vi "MT MSK Mod-Demod.vi"() -> ()   [LabVIEW 2010]
doc: "This example demonstrates the programming of an MSK Modulation Demodulation System."
uses:
  <vilib>/addons/Modulation/Digital/General/MT Generate Bits (Galois, PN Order).vi
  <vilib>/AddOns/Modulation/Digital/General/MT Generate MSK System Parameters.vi
  <vilib>/AddOns/Modulation/Digital/General/MT Apply Matched Filter (MSK).vi
  <vilib>/AddOns/Modulation/Digital/General/MT Align To Ideal Symbols (MSK).vi
  <vilib>/AddOns/Modulation/Digital/General/MT Map MSK Symbols to Bits.vi
  <vilib>/AddOns/Modulation/Digital/Demodulation/MT Calculate BER After Trigger (PN Sequence).vi
  <vilib>/addons/Modulation/niDMT.lvlib
panel:
  in  "autoscale":bool
  out "Constellation Graph, RX (in)":T1(graph)
  out "Recovered Message Bits":i8[](array[numeric])
  in  "Differential Encoding Enable":enum16{"disable", "enable"}(ring)
  in  "Seed In":i32=-1
  out "error out":errorcluster
  in  "stop":bool
  out "BER":dbl format="%.4f"
  in  "PN Sequence Order":i32=9
  in  "Reset? (T)":bool=TRUE
  in  "Eb/N0 (dB)":dbl(slide)=50.0 scale=0.0..100.0
  in  "Symbol Rate (Hz)":dbl=400000.0 format="%.2p"
  in  "Pulse Shaping Filter":T2(ring)=enum."Gaussian"
  in  "MSK Symbols":i32=1000
  in  "Samples per Symbol":i32=16
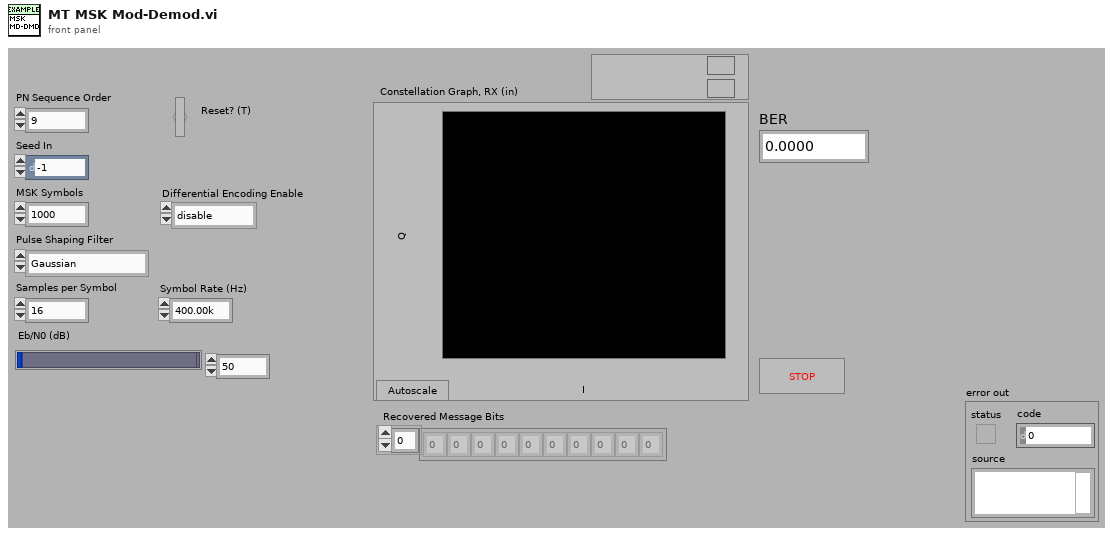
[diagram p1: front panel]
types:
  T1 = cluster{"Decimated Array":dbl[], "Decimated Array":dbl[]}[]
  T2 = enum16{"none", "Raised Cosine", "Root Raised Cos", "Gaussian"}
  T3 = enum16{"FSK", "PSK", "QAM", "MSK", "PAM", "ASK", "CPM"}
  T4 = cluster{"differential encoding enable":enum16{"disable", "enable"}, "samples per symbol (16)":i32}
  T5 = typedef "niAMT.lvlib/Complex Data Waveform.ctl" = cluster{"t0":dbl, "dt":dbl, "Y":cdb[]}
  T6 = cluster{"constellation":dbl[], "oversampled data":dbl[]}[]
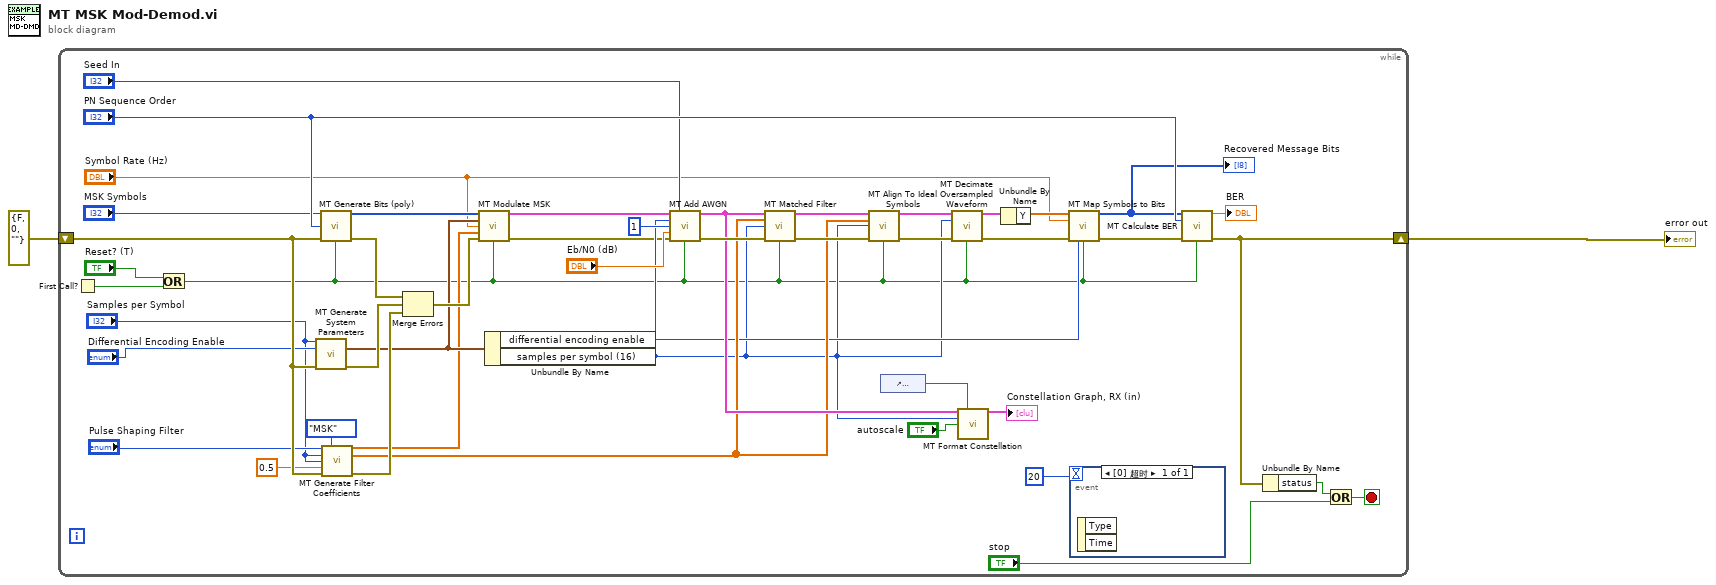
[diagram p0: block diagram]
diagram:
  n1 = while {
    shift-right: [w38] -> w2
    shift-left: errorcluster {"status"=FALSE, "code"=0, "source"=""} ("error out") -> [w49]
    stop <- w37 stop-if-true
    n2 = First Call?() -> (First Call?: T/F=w28:bool)
    n3 = Or(x="Reset? (T)", y=w28) -> (x .or. y?=w6:bool)
    n4 = call-poly <vilib>:"MT Generate System Parameters.vi"("samples per symbol (16)"="Samples per Symbol", "differential encoding enable"="Differential Encoding Enable", "error in (no error)"=w49) -> ("MSK system parameters"=w10:T4, "error out"=w44:errorcluster)  [unwired: 2 in, 9 out]
    n5 = call-poly <vilib>:"MT Generate Bits (poly).vi"("total bits (128)"="MSK Symbols", "PN sequence order (9)"="PN Sequence Order", "error in (no error)"=w49, "reset? (T)"=w6) -> ("output bit stream"=w11:i8[], "error out"=w45:errorcluster)  [unwired: 1 in, 9 out]
    n6 = call <vilib>:"MT Generate Filter Coefficients.vi"("pulse shaping filter (none)"="Pulse Shaping Filter", "modulation type"=T3."MSK", "pulse shaping samples per symbol (16)"="Samples per Symbol", "matched samples per symbol (16)"="Samples per Symbol", "filter parameter"=0.5, "error in (no error)"=w49) -> ("pulse shaping filter coefficients"=w8:dbl[], "matched filter coefficients"=w19:dbl[], "error out"=w43:errorcluster)  [unwired: 1 in, 6 out]
    n7 = Merge Errors(w45, w44, w43) -> (w48:errorcluster)
    n8 = call <vilib>:"MT Modulate MSK.vi"("input bit stream"=w11, "MSK system parameters"=w10, "symbol rate (Hz)"="Symbol Rate (Hz)", "pulse shaping filter coefficients"=w8, "error in (no error)"=w48, "reset? (T)"=w6) -> ("output complex waveform"=w7:T5, "error out"=w5:errorcluster)  [unwired: 1 in, 7 out]
    n9 = Unbundle By Name(w10) -> ("differential encoding enable"=w14:enum16{"disable", "enable"}, "samples per symbol (16)"=w12:i32)
    n10 = call <vilib>:"MT Add AWGN.vi"("input complex waveform"=w7, "samples per symbol (16)"=w12, "bits per symbol (1)"=1, "Eb/N0 (10 dB)"="Eb/N0 (dB)", "error in (no error)"=w5, "seed in (0xFFFFFFFF)"="Seed In", "reset? (T)"=w6) -> ("output complex waveform"=w22:T5, "error out"=w27:errorcluster)  [unwired: 7 out]
    n11 = call-poly <vilib>:"MT Matched Filter.vi"("input complex waveform"=w22, "matched filter coefficients"=w19, "samples per symbol (16)"=w12, "error in (no error)"=w27, "reset? (T)"=w6) -> ("output phase waveform"=w20:cluster{"t0":dbl, "dt":dbl, "Y":dbl[]}, "error out"=w23:errorcluster)  [unwired: 9 out]
    n12 = call-poly <vilib>:"MT Align To Ideal Symbols.vi"("input phase waveform"=w20, "matched filter coefficients"=w19, "samples per symbol (16)"=w12, "error in (no error)"=w23, "reset? (T)"=w6) -> ("output phase waveform"=w17:cluster{"t0":dbl, "dt":dbl, "Y":dbl[]}, "error out"=w21:errorcluster)  [unwired: 9 out]
    n13 = control-ref of="Constellation Graph, RX (in)"() -> (w30:refnum<vi>)
    n14 = call <vilib>:"MT Decimate Oversampled Waveform.vi"("input complex waveform"=w17, "decimation factor"=w12, "error in (no error)"=w21, "reset? (T)"=w6) -> ("output complex waveform"=w16:T5, "error out"=w18:errorcluster)  [unwired: 1 in, 9 out]
    n15 = call <vilib>:"MT Format Constellation.vi"("waveform"=w22, "constellation reference"=w30, "samples per symbol"=w12, "autoscale"="autoscale") -> ("constellation graph"=→"Constellation Graph, RX (in)":T6)  [unwired: 1 in, 10 out]
    n16 = Unbundle By Name(w16) -> ("Y"=w15:cdb[])
    n17 = call-poly <vilib>:"MT Map Symbols to Bits.vi"("symbols"=w15, "symbol rate"="Symbol Rate (Hz)", "error in (no error)"=w18, "differential encoding enable"=w14, "reset? (T)"=w6) -> ("output bit stream"=w25:i8[], "error out"=w24:errorcluster)  [unwired: 9 out]
    "Recovered Message Bits" <- w25
    n18 = event shown="[0] 超时" {
      selector: _ -> [_]
      dyn-events: _ -> [_]
      timeout: 20 -> [_]
      event Timeout {
        n19 = event-data() -> ()  [unwired: 3 out]
      }
    }
    n20 = call-poly <vilib>:"MT Calculate BER.vi"("input bit stream"=w25, "PN sequence order (9)"="PN Sequence Order", "error in (no error)"=w24, "reset? (T)"=w6) -> ("BER"=→"BER":dbl, "error out"=w38:errorcluster)  [unwired: 2 in, 8 out]
    n21 = Unbundle By Name(w38) -> ("status"=w36:bool)
    n22 = Or(x=w36, y="stop") -> (x .or. y?=w37:bool)
  }
  "error out" <- w2
